vi "Actor Core.vi"(8 "error in":errorcluster, 11 "Measure Object in":refnum<class "Resonance Detector.lvclass">) -> (0 "error out":errorcluster, 3 "Actor out":refnum<class "Actor.lvclass">)   [LabVIEW 2018, in "Resonance Detector.lvclass"]
doc: "Line Detector module finds amplitude peaks in spectrum file and fits complex Lorentzian around peaks"
uses:
  Resonance Detector.lvclass
  C:/github/LabActor/Template Module/Template Module.lvclass
  C:/Program Files/National Instruments/LabVIEW 2018/vi.lib/ActorFramework/Actor/Actor.lvclass
  <vilib>/ActorFramework/Actor/Actor.lvclass
  Resonance Detector Configuration.ctl
  Resonance Detector.lvclass/Resonance Detector.ctl
  Template Module/Template Module.lvclass/Template Module.ctl
  <vilib>/ActorFramework/Actor/Actor.lvclass/Actor.ctl
  <vilib>/ActorFramework/Message Enqueuer/Message Enqueuer.lvclass/Message Enqueuer.ctl
  NHMFL_Core/Libraries/Instruments/Results/File Path Result/File Path Result.lvclass
  C:/github/NHMFL_Core/Libraries/Instruments/Results/Acquired Result/Acquired Result.lvclass
  Process Object Messages/Process Result Msg/Process Result Msg.lvclass/Process Result Msg.ctl
  <vilib>/Utility/sysdir.llb/System Directory Type.ctl
  Template Module/Read stop event.vi
  <vilib>/ActorFramework/Message Enqueuer/Init from Existing Queue.vi
  <vilib>/ActorFramework/Message Enqueuer/Enqueue.vi
  Process Object Messages/Process Result Msg/Process Result Msg.lvclass
  C:/Program Files/National Instruments/LabVIEW 2018/vi.lib/ActorFramework/Message/Message.lvclass
  <vilib>/ActorFramework/Message Priority Queue/Priority Enqueue.vi
  <vilib>/Utility/file.llb/Write Delimited Spreadsheet (DBL).vi
  <vilib>/Utility/file.llb/Read Delimited Spreadsheet (DBL).vi
  Process Object/Process Object.lvclass
  <vilib>/ActorFramework/Message Enqueuer/Message Enqueuer.lvclass
panel:
  in  "Best fit results":dbl[][](array[numeric]) format="%#_10p"
  in  "Plot Tab Control":enum32{"Spectrum fit", "Peak finder"}(tab)
  in  "Save table":bool
  in  "Load table":bool
  out "Spectrum fit":cluster{dbl[], dbl[]}[](graph)
  out "Peak Plot":cluster{"Ramp Pattern":dbl[], "X":dbl[]}[](graph)
  out "Name":string
  in  "Re-process":bool
  in  "Configuration":T1={"Peak width guess"=500.0, "Background removal"=enum."High-pass", "Smoothing"=enum."Low-pass", "Smooth window"=200.0, "Relative threshold"=0.2, "Finder algorithm"=enum."Wavelet", "Bgd window"=50000.0, "Spectrum recorder module name"="Spectrum Recorder", "Fit window"=1000.0, "Initial fit guess"=enum."Peak finder", "Follow\npeaks"=FALSE, "Re-sample"=nan} {"Re-sample" format="%#_6pHz"; "Fit window" format="%#_6pHz"; "Bgd window" format="%#_6pHz"; "Smooth window" format="%#_6pHz"; "Peak width guess" format="%#_6pHz"}
  in  "Input file":path
  # "Follow"
  # "f0    |    g    |   A   |  q   |   Xbg  |  Ybg |mask"
  # "Peak finder config"
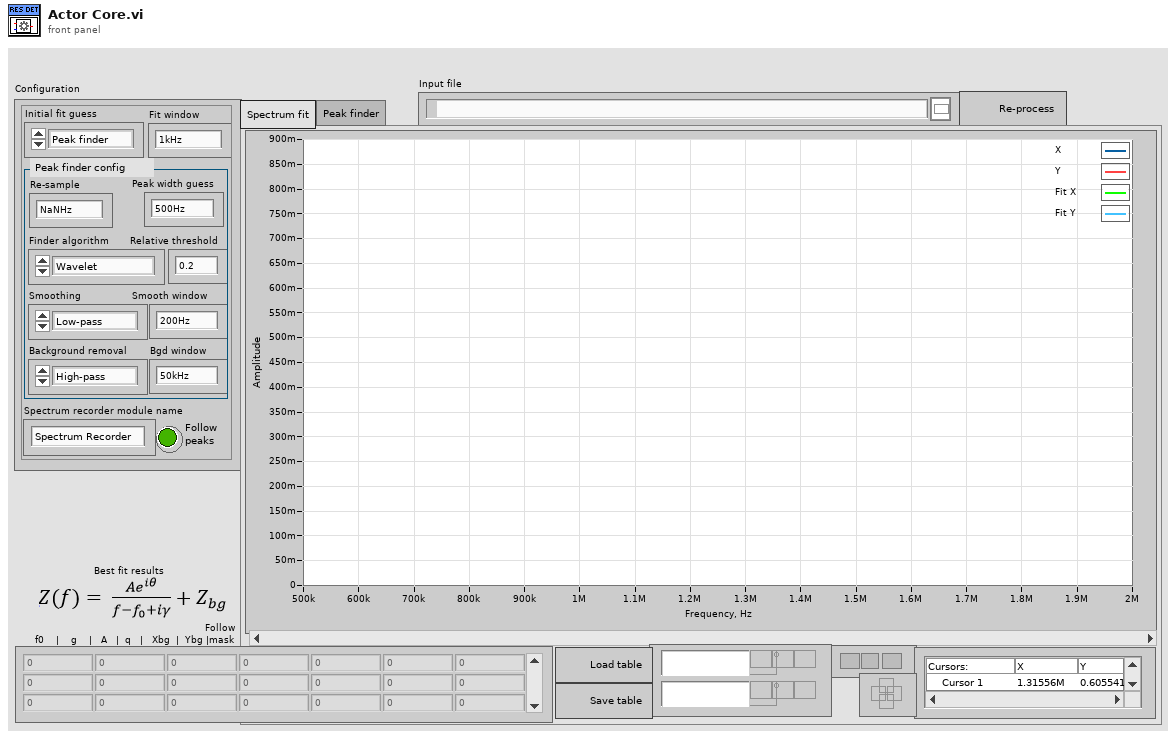
[diagram p1: front panel]
types:
  T1 = typedef "Resonance Detector Configuration.ctl" = cluster{"Peak width guess":dbl, "Background removal":enum16{"NONE", "High-pass", "Detrend"}, "Smoothing":enum16{"NONE", "Low-pass", "Denoise"}, "Smooth window":dbl, "Relative threshold":dbl, "Finder algorithm":enum16{"Basic", "Wavelet", "Wavelet+detrend"}, "Bgd window":dbl, "Spectrum recorder module name":string, "Fit window":dbl, "Initial fit guess":enum16{"Peak finder", "Last fit"}, "Follow\npeaks":bool, "Re-sample":dbl}
  T2 = typedef "System Directory Type.ctl" = i32
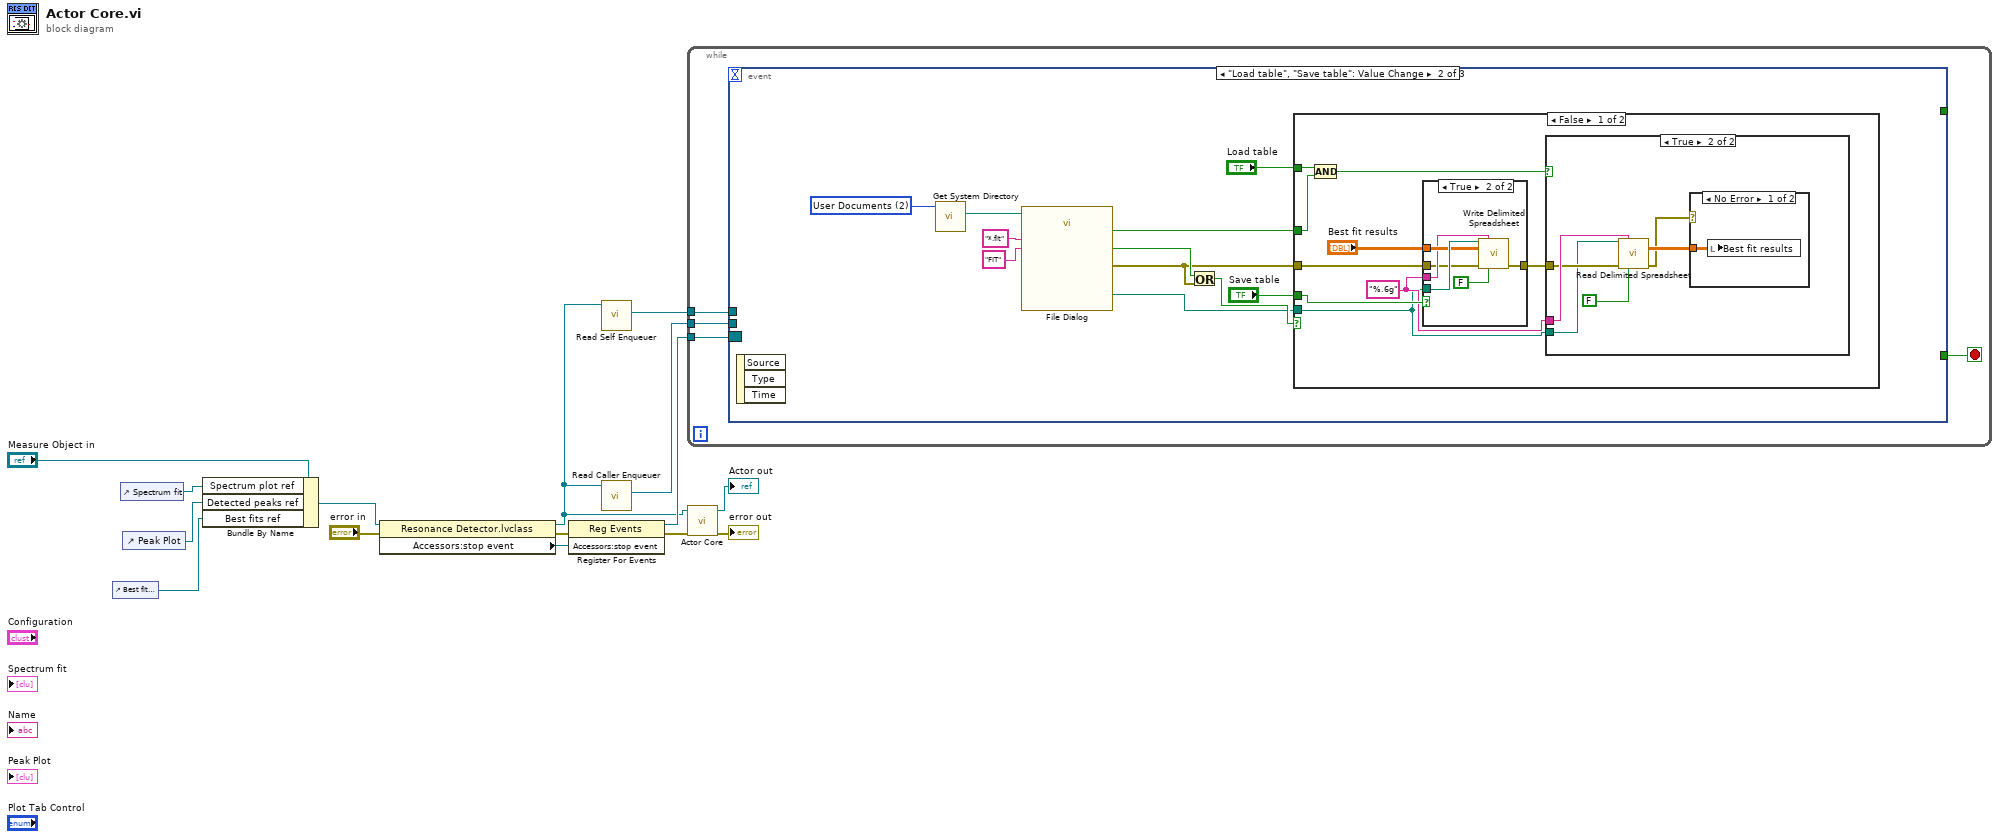
[diagram p0: block diagram]
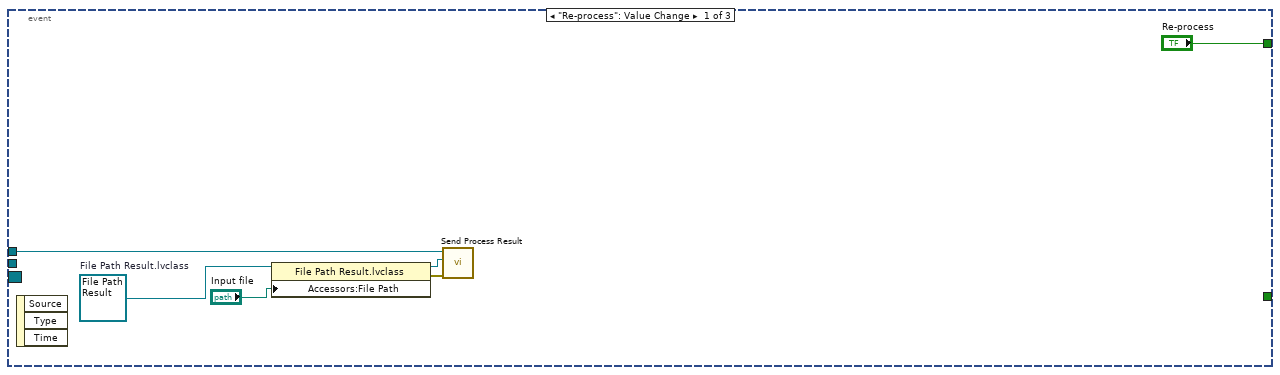
[diagram p2: hidden frame]
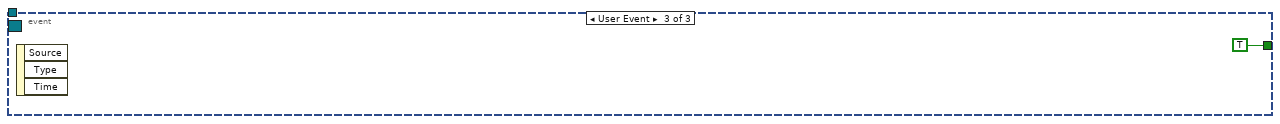
[diagram p7: hidden frame]
diagram:
  n1 = control-ref of="Best fit results"() -> (w4:refnum<vi>)
  n2 = control-ref of="Spectrum fit"() -> (w6:refnum<vi>)
  n3 = control-ref of="Peak Plot"() -> (w5:refnum<vi>)
  n4 = Bundle By Name(cluster="Measure Object in", "Spectrum plot ref"=w6, "Detected peaks ref"=w5, "Best fits ref"=w4) -> (w7:refnum<class "Resonance Detector.lvclass">)
  n5 = property class="Resonance Detector.lvclass"(reference=w7, error in="error in") -> (reference out=w1:refnum<class "Resonance Detector.lvclass">, error out=w11:errorcluster, "Accessors:stop event"=w13:refnum<user-event>)
  n6 = register-events(error in=w11, w13) -> (reference out=w12:refnum<event-registration>, error out=w3:errorcluster)  [unwired: 1 in]
  n7 = call <vilib>:"Read Self Enqueuer.vi"("Actor"=w1) -> ("Self Enqueuer"=w10:refnum<class "Message Enqueuer.lvclass">)  [unwired: 10 in]
  n8 = call <vilib>:"Read Caller Enqueuer.vi"("Actor"=w1) -> ("Caller Enqueuer"=w2:refnum<class "Message Enqueuer.lvclass">)  [unwired: 10 in]
  n9 = while {
    tunnel: w12 -> [w19]
    tunnel: w10 -> [w17]
    tunnel: w2 -> [w16]
    stop <- w18 stop-if-true
    n10 = event shown="[1] \"Load table\", \"Save table\": Value Change" {
      selector: w19 -> [_ _ _]
      dyn-events: _ -> [_ _ _]
      timeout: _ -> [_ _ _]
      tunnel: [_ _ TRUE] -> w18
      tunnel: w17 -> [w25 _ _]
      tunnel: ["Re-process" _ _] -> _
      tunnel: w16 -> [_ _ _]
      event "Re-process": Value Change {
        w24 = refnum<class "File Path Result.lvclass"> refnum  # File Path Result.lvclass
        n11 = event-data() -> ()  [unwired: 1 in, 3 out]
        n12 = property class="File Path Result.lvclass"(reference=w24, "Accessors:File Path"="Input file") -> (reference out=w23:refnum<class "File Path Result.lvclass">, error out=w22:errorcluster)  [unwired: 1 in]
        n13 = call "Send Process Result.vi"("error in (no error)"=w22, "Result in"=w23, "Message Enqueuer"=w25) -> ()  [unwired: 7 in, 2 out]
      }
      event "Load table", "Save table": Value Change {
        w35 = T2 2 items=["User Home"=0, "User Desktop"=1, "User Documents"=2, "User Application Data"=3, "User Preferences"=4, "User Temporary"=5, "Public Documents"=6, "Public Application Data"=7, "Public Preferences"=8, "Public Cache"=13, "System Core Libraries"=9, "System Installed Libraries"=10, "Application Files"=11, "Boot Volume Root"=12] ("system directory type")
        n14 = event-data() -> ()  [unwired: 1 in, 3 out]
        n15 = call <vilib>:"Get System Directory.vi"("system directory type"=w35) -> ("system directory"=w36:path)  [unwired: 10 in]
        n16 = call "File Dialog"("start path"=w36, "pattern (all files)"="*.fit", "pattern label"="FIT") -> ("selected path"=w30:path, "exists"=w31:bool, "cancelled"=w32:bool, "error out"=w26:errorcluster)  [unwired: 9 in]
        n17 = Or(x=w32, y=w26) -> (x .or. y?=w33:bool)
        n18 = case shown="False" w33 {
          tunnel: w31 -> [w44 _]
          tunnel: w30 -> [w38 _]
          tunnel: "Load table" -> [w41 _]
          tunnel: "Save table" -> [w40 _]
          tunnel: w26 -> [w37 _]
          frame False {
            w39 = "%.6g" ("format (%.3f)")
            n19 = And(x=w41, y=w44) -> (x .and. y?=w45:bool)
            n20 = case shown="True" w40 {
              tunnel: "Best fit results" -> [_ w51]
              tunnel: [w46 w50] -> w42
              tunnel: w38 -> [_ w52]
              tunnel: w39 -> [_ w49]
              tunnel: w37 -> [w46 w47]
              frame False {
              }
              frame True {
                n21 = call-poly <vilib>:"Write Delimited Spreadsheet.vi"("file path (dialog if empty)"=w52, "format (%.3f)"=w49, "2D data"=w51, "error in (no error)"=w47, "transpose? (no:F)"=FALSE) -> ("error out"=w50:errorcluster)  [unwired: 9 in, 1 out]
              }
            }
            n22 = case shown="True" w45 {
              tunnel: w42 -> [_ w57]
              tunnel: w39 -> [_ w58]
              tunnel: w38 -> [_ w56]
              frame False {
              }
              frame True {
                n23 = call-poly <vilib>:"Read Delimited Spreadsheet.vi"("file path (dialog if empty)"=w56, "format (%.3f)"=w58, "error in (no error)"=w57, "transpose? (F)"=FALSE) -> ("all rows"=w54:dbl[][], "error out"=w53:errorcluster)  [unwired: 6 in, 4 out]
                n24 = case shown="No Error" w53 {
                  tunnel: w54 -> [w59 _]
                  frame No Error {
                    n25 = local write "Best fit results"(w59) -> ()
                  }
                  frame Error {
                  }
                }
              }
            }
          }
          frame True {
          }
        }
      }
      event User Event {
        n26 = event-data() -> ()  [unwired: 1 in, 3 out]
      }
    }
  }
  n27 = call-parent "Actor Core.vi"("error in"=w3, "Measure Object in"=w1) -> ("error out"=→"error out":errorcluster, "Actor out"=→"Actor out":refnum<class "Actor.lvclass">)  [unwired: 8 in]
